vi "Get Motor Inertia.vi"(8 "error in (no error)":errorcluster, 11 "Link in":refnum<class "NI_Robotics_Link.lvclass">) -> (0 "error out":errorcluster, 2 "Motor Inertia":dbl, 3 "Link out":refnum<class "NI_Robotics_Link.lvclass">)   [LabVIEW 2017, in "NI_Robotics_Link.lvclass"]
uses:
  <vilib>/robotics/Kinematics/Link/NI_Robotics_Link.lvclass
  <vilib>/robotics/Kinematics/Link/NI_Robotics_Link.lvclass/NI_Robotics_Link.ctl
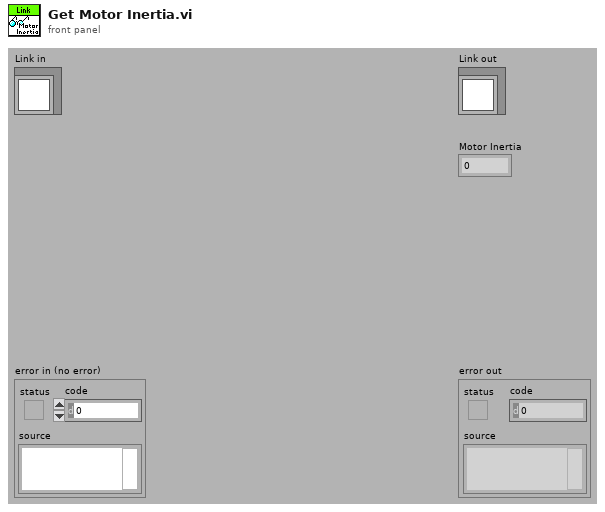
[diagram p1: front panel]
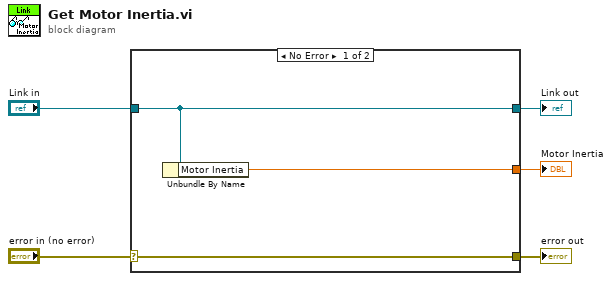
[diagram p0: block diagram]
diagram:
  n1 = case shown="No Error" "error in (no error)" {
    selector: "error in (no error)" -> [w8 w9]
    tunnel: [w8 w9] -> w4
    tunnel: [w7 w10] -> w2
    tunnel: "Link in" -> [w7 w10]
    tunnel: [w6 _] -> w1
    frame No Error {
      n2 = Unbundle By Name(w7) -> ("Motor Inertia"=w6:dbl)
    }
    frame Error {
    }
  }
  "error out" <- w4
  "Link out" <- w2
  "Motor Inertia" <- w1
